vi "IS Set Access Key.vi"(0 "HTTP Client Handle in":T1, 1 "Access Key":string, 3 "error in (no error)":errorcluster) -> (7 "HTTP Client Handle out":T1, 10 "error out":errorcluster)   [LabVIEW 2013]
uses:
  <vilib>/httpClient/LabVIEWHTTPClient.lvlib
  <vilib>/httpClient/ClientHandle.ctl
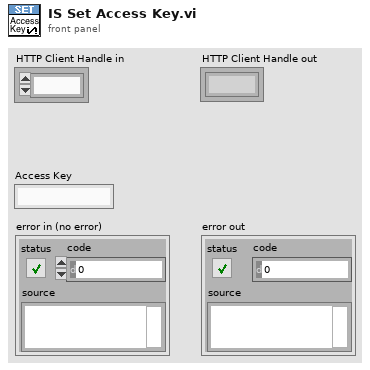
[diagram p1: front panel]
types:
  T1 = typedef "LabVIEWHTTPClient.lvlib/ClientHandle.ctl" = refnum<k1>
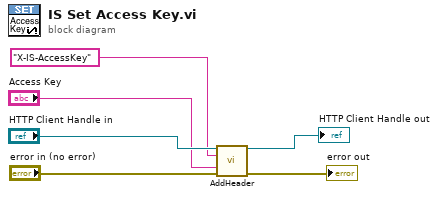
[diagram p0: block diagram]
diagram:
  n1 = call <vilib>:"AddHeader.vi"("client handle"="HTTP Client Handle in", "header"="X-IS-AccessKey" ("String"), "value"="Access Key", "error in (no error)"="error in (no error)") -> ("client handle out"=→"HTTP Client Handle out":T1, "error out"=→"error out":errorcluster)  [unwired: 10 in]
